vi "config-Motors-v2.vi"(8 "error in":errorcluster, 10 "Acc":dbl, 11 "Velocity":sgl) -> (0 "error out":errorcluster)   [LabVIEW 2021]
doc: "André Romero - 2023\nandretec@ifsc.usp.br\nIFSC - USP"
uses:
  Global Motors.vi
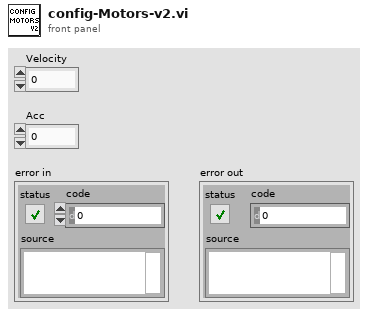
[diagram p1: front panel]
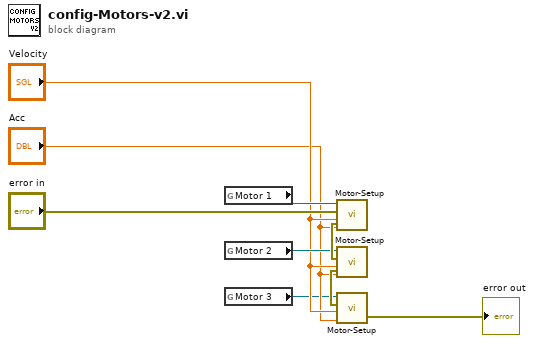
[diagram p0: block diagram]
diagram:
  n1 = global read "Global Motors.vi" "Motor 1"() -> (w6:refnum<k7>)
  n2 = global read "Global Motors.vi" "Motor 2"() -> (w7:refnum<k7>)
  n3 = global read "Global Motors.vi" "Motor 3"() -> (w2:refnum<k7>)
  n4 = call "Motor-Setup.vi"("Acc"="Acc", "Velocidade"="Velocity", "error"="error in", "MG17Motor A"=w6) -> ("error out"=w9:errorcluster)  [unwired: 1 out]
  n5 = call "Motor-Setup.vi"("Acc"="Acc", "Velocidade"="Velocity", "error"=w9, "MG17Motor A"=w7) -> ("error out"=w5:errorcluster)  [unwired: 1 out]
  n6 = call "Motor-Setup.vi"("Acc"="Acc", "Velocidade"="Velocity", "error"=w5, "MG17Motor A"=w2) -> ("error out"=→"error out":errorcluster)  [unwired: 1 out]
